vi "XML.Generate.vi"(8 "error in":errorcluster, 9 "Computer ID":string, 10 "Clusters refs":refnum<vi>[](array[refnum]), 11 "XML file path":path=path "C:/Projects/TM-OS/trunk/Design/XML_HW_config2.xml") -> (0 "error out":errorcluster)   [LabVIEW 2019, in "Tools.lvlib"]
uses:
  Tools.lvlib
  LibXML/LibXML.lvlib
panel:
  in  "Root name":string="HWConfigFile"
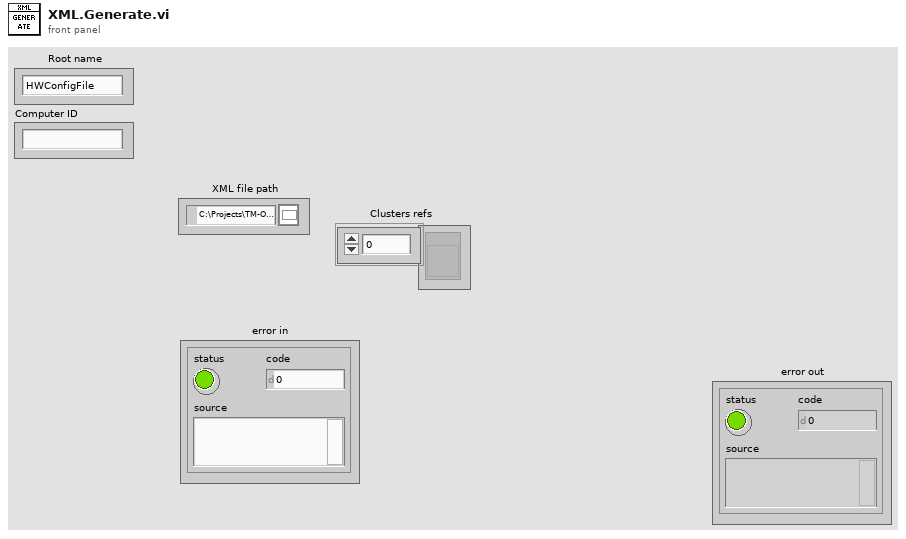
[diagram p1: front panel]
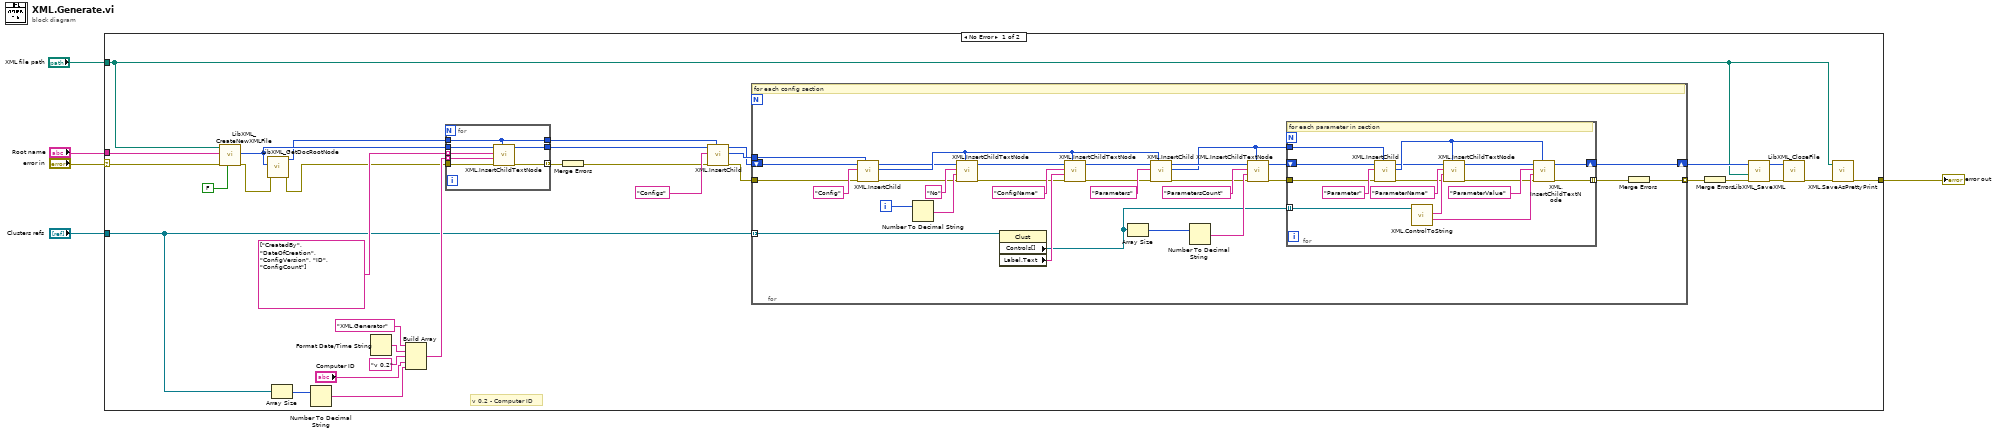
[diagram p0: block diagram]
diagram:
  n1 = case shown="No Error" "error in" {
    selector: "error in" -> [w17 w91]
    tunnel: "Clusters refs" -> [w32 _]
    tunnel: [w20 w91] -> w3
    tunnel: "Root name" -> [w16 _]
    tunnel: "XML file path" -> [w6 _]
    frame No Error {
      # "v 0.2 - Computer ID"
      n2 = call "LibXML_CreateNewXMLFile.vi"("Assign this Schema"=FALSE, "error in"=w17, "Root element name"=w16, "file path"=w6) -> ("error out"=w14:errorcluster, "new doc out"=w13:u32)  [unwired: 5 in, 1 out]
      n3 = call "LibXML_GetDocRootNode.vi"("error in"=w14, "doc"=w13) -> ("error out"=w15:errorcluster, "root node out"=w12:u32)  [unwired: 8 in]
      n4 = Array Size(array=w32) -> (size(s)=w31:i32)
      n5 = Number To Decimal String(number=w31) -> (decimal integer string=w30:string)  [unwired: 1 in]
      n6 = Format Date/Time String() -> (date/time string=w34:string)  [unwired: 3 in]
      n7 = Build Array("XML.Generator" ("Tag Name"), w34, "v 0.2" ("element"), "Computer ID", w30) -> (w35:string[])
      n8 = for {
        tunnel: string[] ["CreatedBy", "DateOfCreation", "ConfigVersion", "ID", "ConfigCount"] -> [w44] mode=indexing
        tunnel: w13 -> [w41]
        tunnel: w12 -> [w40]
        tunnel: w35 -> [w43] mode=indexing
        tunnel: [w42] -> w27
        tunnel: [w40] -> w25
        tunnel: w15 -> [w39]
        tunnel: [w38] -> w24 mode=indexing
        n9 = call "XML.InsertChildTextNode.vi"("parent"=w40, "error in"=w39, "text"=w43, "name"=w44, "doc"=w41) -> ("error out"=w38:errorcluster, "doc out"=w42:u32)  [unwired: 5 in]
      }
      n10 = Merge Errors(w24) -> (w23:errorcluster)
      n11 = call "XML.InsertChild.vi"("parent"=w25, "error in"=w23, "name"="Configs" ("Tag Name"), "doc"=w27) -> ("error out"=w22:errorcluster, "new node"=w29:u32, "doc out"=w26:u32)  [unwired: 5 in]
      n12 = for {
        tunnel: w32 -> [w54] mode=indexing
        tunnel: w29 -> [w73]
        shift-right: [w71] -> w8
        shift-left: w26 -> [w72]
        tunnel: w22 -> [w52]
        tunnel: [w45] -> w21 mode=indexing
        i -> [w74]
        # "for each config section"
        n13 = call "XML.InsertChild.vi"("parent"=w73, "error in"=w52, "name"="Config" ("Tag Name"), "doc"=w72) -> ("error out"=w51:errorcluster, "new node"=w61:u32, "doc out"=w58:u32)  [unwired: 5 in]
        n14 = Number To Decimal String(number=w74) -> (decimal integer string=w69:string)  [unwired: 1 in]
        n15 = call "XML.InsertChildTextNode.vi"("parent"=w61, "error in"=w51, "text"=w69, "name"="No" ("Tag Name"), "doc"=w58) -> ("error out"=w50:errorcluster, "doc out"=w57:u32)  [unwired: 5 in]
        n16 = property class="Clust"(reference=w54) -> ("Controls[]"=w53:refnum<vi>[], "Label.Text"=w67:string)  [unwired: 1 in, 2 out]
        n17 = call "XML.InsertChildTextNode.vi"("parent"=w61, "error in"=w50, "text"=w67, "name"="ConfigName", "doc"=w57) -> ("error out"=w49:errorcluster, "doc out"=w59:u32)  [unwired: 5 in]
        n18 = Array Size(array=w53) -> (size(s)=w65:i32)
        n19 = call "XML.InsertChild.vi"("parent"=w61, "error in"=w49, "name"="Parameters" ("Tag Name"), "doc"=w59) -> ("error out"=w48:errorcluster, "new node"=w55:u32, "doc out"=w60:u32)  [unwired: 5 in]
        n20 = Number To Decimal String(number=w65) -> (decimal integer string=w64:string)  [unwired: 1 in]
        n21 = call "XML.InsertChildTextNode.vi"("parent"=w55, "error in"=w48, "text"=w64, "name"="ParametersCount", "doc"=w60) -> ("error out"=w47:errorcluster, "doc out"=w56:u32)  [unwired: 5 in]
        n22 = for {
          tunnel: w55 -> [w87]
          shift-right: [w80] -> w71
          shift-left: w56 -> [w86]
          tunnel: w53 -> [w79] mode=indexing
          tunnel: w47 -> [w78]
          tunnel: [w75] -> w46 mode=indexing
          # "for each parameter in section"
          n23 = call "XML.InsertChild.vi"("parent"=w87, "error in"=w78, "name"="Parameter" ("Tag Name"), "doc"=w86) -> ("error out"=w77:errorcluster, "new node"=w85:u32, "doc out"=w84:u32)  [unwired: 5 in]
          n24 = call "XML.ControlToString.vi"("control ref in"=w79) -> ("string value"=w82:string, "label"=w81:string)  [unwired: 7 in, 2 out]
          n25 = call "XML.InsertChildTextNode.vi"("parent"=w85, "error in"=w77, "text"=w81, "name"="ParameterName", "doc"=w84) -> ("error out"=w76:errorcluster, "doc out"=w83:u32)  [unwired: 5 in]
          n26 = call "XML.InsertChildTextNode.vi"("parent"=w85, "error in"=w76, "text"=w82, "name"="ParameterValue", "doc"=w83) -> ("error out"=w75:errorcluster, "doc out"=w80:u32)  [unwired: 5 in]
        }
        n27 = Merge Errors(w46) -> (w45:errorcluster)
      }
      n28 = Merge Errors(w21) -> (w11:errorcluster)
      n29 = call "LibXML_SaveXML.vi"("error in"=w11, "file path (dialog if empty)"=w6, "doc"=w8) -> ("error out"=w10:errorcluster, "doc copy out"=w9:u32)  [unwired: 6 in, 1 out]
      n30 = call "LibXML_CloseFile.vi"("error in"=w10, "doc"=w9) -> ("error out"=w7:errorcluster)  [unwired: 9 in]
      n31 = call "XML.SaveAsPrettyPrint.vi"("error in (no error)"=w7, "XML file path"=w6) -> ("error out"=w20:errorcluster)  [unwired: 9 in]
    }
    frame Error {
    }
  }
  "error out" <- w3
